vi "VerifyMove.vi"(6 "Position in":T4, 9 "Direction in":T1=enum."N", 10 "Desired Action":T3, 11 "Map DVR":T2) -> (1 "Direction":T1, 2 "Action":T3, 3 "Map DVR out":T2, 4 "Accepted?":bool)   [LabVIEW 2020, in "Atom.lvclass"]
uses:
  Atom.lvclass
  Type Defs/Action Enum.ctl
  Type Defs/Direction Enum.ctl
  Common/Map DVR.ctl
  Common/Location Data.ctl
  Common/Position.ctl
  SubVIs/Read-Only Globals.vi
  Square/Board Size.vi
  SubVIs/Globals (private).vi
  Type Defs/SB Type Defs.lvlib
  Common/Common.lvlib
  Square/Square.lvclass
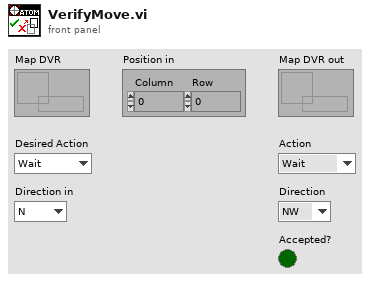
[diagram p1: front panel]
types:
  T1 = typedef "SB Type Defs.lvlib/Direction Enum.ctl" = enum16{"NW", "N", "NE", "E", "SE", "S", "SW", "W"}
  T2 = typedef "Common.lvlib/Map DVR.ctl" = refnum<data-value>
  T3 = typedef "SB Type Defs.lvlib/Action Enum.ctl" = enum16{"Wait", "Move", "Attack", "Replicate"}
  T4 = typedef "Common.lvlib/Position.ctl" = cluster{"Column":i32, "Row":i32}
  T5 = typedef "Common.lvlib/Location Data.ctl" = cluster{"Location State":enum16{"Empty", "Enemy", "Attacked", "Occupied"}, "Round Updated":i32}
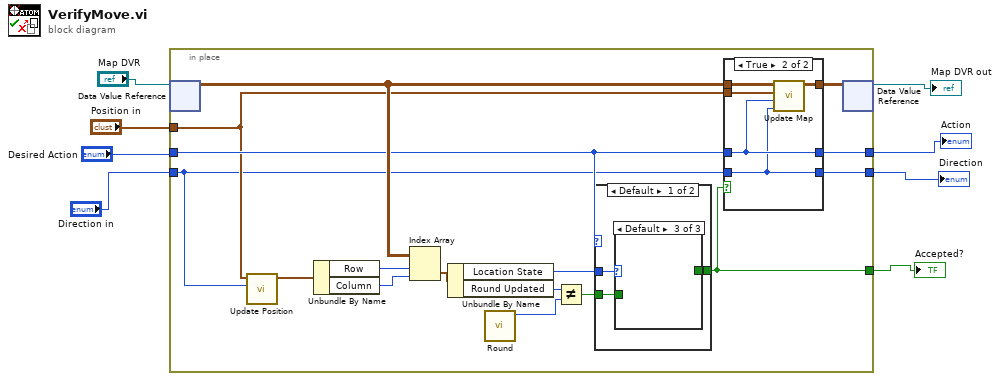
[diagram p0: block diagram]
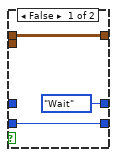
[diagram p2: hidden frame]
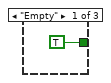
[diagram p3: hidden frame]
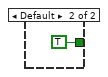
[diagram p6: hidden frame]
diagram:
  n1 = in-place {
    in-place-border: [w18] -> w3
    in-place-border: "Position in" -> [w16]
    in-place-border: [w22] -> w2
    in-place-border: "Desired Action" -> [w17]
    in-place-border: [w21] -> w4
    in-place-border: "Direction in" -> [w15]
    n2 = in-place-dvr #1("Map DVR") -> (w24:T5[][])  [unwired: 1 out]
    n3 = call "Update Position.vi"("Direction"=w15, "Position in"=w16) -> ("Position out"=w14:T4)  [unwired: 9 in]
    n4 = Unbundle By Name(w14) -> ("Row"=w13:i32, "Column"=w12:i32)
    n5 = Index Array(array=w24, index (row)=w13, index (col)=w12) -> (element=w20:T5)
    n6 = Unbundle By Name(w20) -> ("Location State"=w19:enum16{"Empty", "Enemy", "Attacked", "Occupied"}, "Round Updated"=w11:i32)
    n7 = call "Round.vi"() -> ("Round"=w9:i32)  [unwired: 11 in]
    n8 = Not Equal?(x=w11, y=w9) -> (x != y?=w10:bool)
    n9 = case shown="Default" w17 {
      tunnel: [w35 w39] -> w21
      tunnel: w19 -> [w34 w38]
      tunnel: w10 -> [w33 _]
      frame Default {
        n10 = case shown="Default" w34 {
          tunnel: [TRUE w37 _] -> w35
          tunnel: w33 -> [_ w37 _]
          frame "Empty" {
          }
          frame "Attacked" {
          }
          frame Default {
          }
        }
      }
      frame "Attack" {
        n11 = case shown="\"Occupied\"" w38 {
          tunnel: [_ TRUE] -> w39
          frame "Occupied" {
          }
          frame Default {
          }
        }
      }
    }
    n12 = case shown="True" w21 {
      tunnel: w15 -> [w26 w28]
      tunnel: w24 -> [w27 w32]
      tunnel: [w27 w31] -> w23
      tunnel: w16 -> [_ w30]
      tunnel: [w26 w28] -> w18
      tunnel: [Action_Enum."Wait" ("Desired Action") w29] -> w22
      tunnel: w17 -> [_ w29]
      frame False {
      }
      frame True {
        n13 = call "Update Map.vi"("Direction"=w28, "Action"=w29, "Old Position"=w30, "Map in"=w32) -> ("Map out"=w31:T5[][])  [unwired: 7 in]
      }
    }
    n14 = in-place-dvr #1(w23) -> (→"Map DVR out":T2)  [unwired: 1 out]
  }
  "Action" <- w2
  "Direction" <- w3
  "Accepted?" <- w4
